vi "SaveBarcodeString.vi"(3 "error in":errorcluster, 5 "String":string) -> (0 "error out":errorcluster)   [LabVIEW 2024]
uses:
  416b9271-cb34-4707-914d-eb77757e1ff1.vi
panel:
  out "cnt. Barcodes":i32
  out "Barcode array":string[](array[string])
  out "array":string[][](array[string])
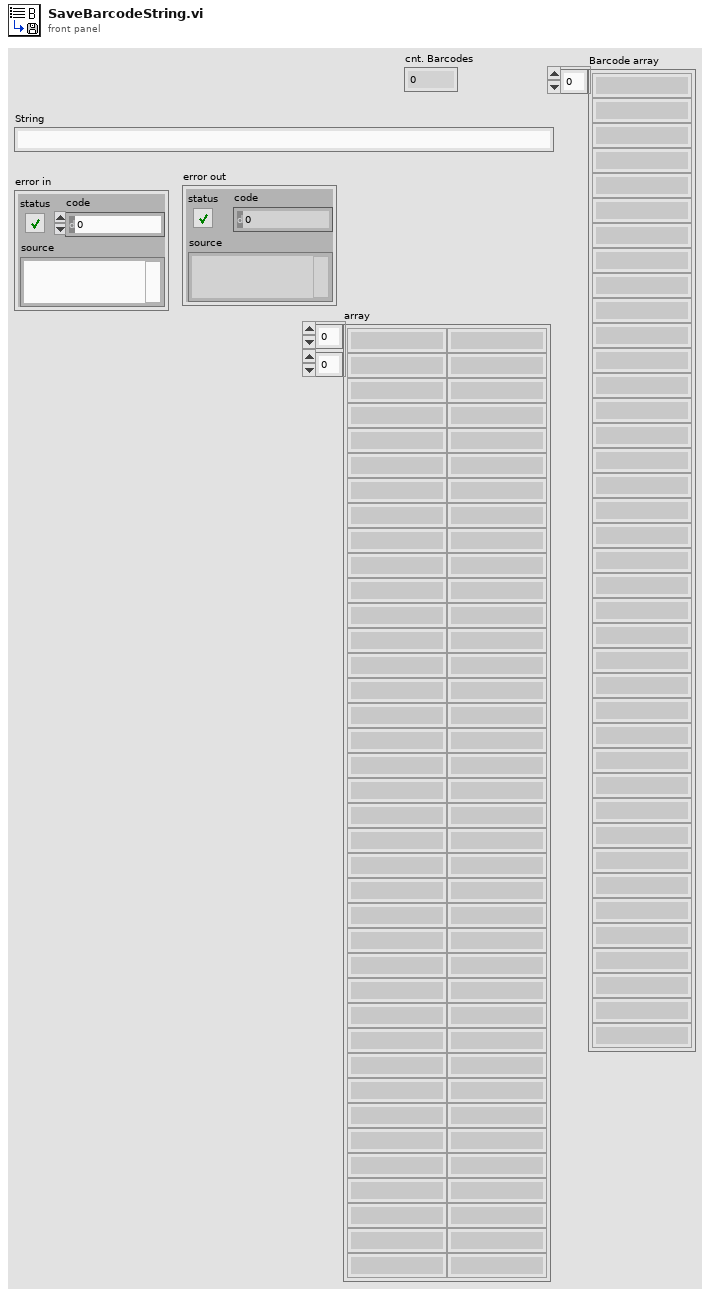
[diagram p1: front panel]
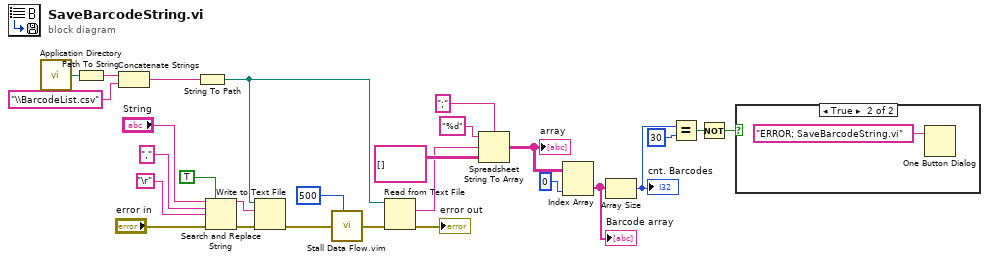
[diagram p0: block diagram]
diagram:
  n1 = call <vilib>:"Application Directory.vi"() -> ("Application Directory"=w27:path)
  n2 = Path To String(path=w27) -> (string=w26:string)
  n3 = Concatenate Strings(w26, "\\BarcodeList.csv" ("string")) -> (w25:string)
  n4 = String To Path(string=w25) -> (path=w6:path)
  n5 = Search and Replace String(replace all?=TRUE ("replace all? (F)"), input string="String", search string=",", replace string="\r", error in="error in") -> (result string=w22:string, error out=w18:errorcluster)  [unwired: 3 in, 2 out]
  n6 = Write to Text File(file (use dialog)=w6, text=w22, error in=w18) -> (error out=w5:errorcluster)  [unwired: 1 in, 2 out]
  n7 = call "Stall Data Flow.vim"("value in"=w5, "milliseconds to wait"=u32 500) -> ("value out"=w4:errorcluster)  [unwired: 1 out]
  n8 = Read from Text File(file (use dialog)=w6, error in=w4) -> (text=w13:string, error out=→"error out":errorcluster)  [unwired: 2 in, 2 out]
  n9 = Spreadsheet String To Array(delimiter (Tab)=";", format string="%d", spreadsheet string=w13, array type (2D Dbl)=string[][] []) -> (array=w12:string[][])
  "array" <- w12
  n10 = Index Array(array=w12, index (col)=0 ("disabled index (col)")) -> (element=w10:string[])  [unwired: 1 in]
  "Barcode array" <- w10
  n11 = Array Size(array=w10) -> (size(s)=w8:i32)
  "cnt. Barcodes" <- w8
  n12 = Equal?(x=w8, y=30) -> (x = y?=w7:bool)
  n13 = Not(x=w7) -> (.not. x?=w1:bool)
  n14 = case shown="True" w1 {
    frame False {
    }
    frame True {
      n15 = One Button Dialog(message="ERROR; SaveBarcodeString.vi" ("string")) -> ()  [unwired: 1 in, 1 out]
    }
  }
